vi "Confirm State Test.vi"(0 "GEA2 Reference In":refnum<k24>, 5 "Standalone?":bool, 7 "State":T1, 11 "Error In":errorcluster) -> (4 "GEA2 Reference Out":refnum<k24>, 6 "Pass/Fail?":bool, 15 "Error Out":errorcluster)   [LabVIEW 2016, in "Centauro.lvlib"]
uses:
  Projects/Centauro.lvlib
  Q:/Common/DLLs/GEA3/GeaCommunication.dll
  Common/DLLs/GEA3/GeaCommunication.dll
  type defs/Machine State.ctl
  Common/LabVIEW GEA2 Toolkit/LabVIEW_GEA2_Toolkit.lvlibp/type defs/Source_Destination.ctl
  Common/LabVIEW GEA2 Toolkit/LabVIEW_GEA2_Toolkit.lvlibp/type defs/ERD Read Data In.ctl
  Common/LabVIEW GEA2 Toolkit/LabVIEW_GEA2_Toolkit.lvlibp/type defs/Data Type.ctl
  Common/LabVIEW GEA2 Toolkit/LabVIEW_GEA2_Toolkit.lvlibp
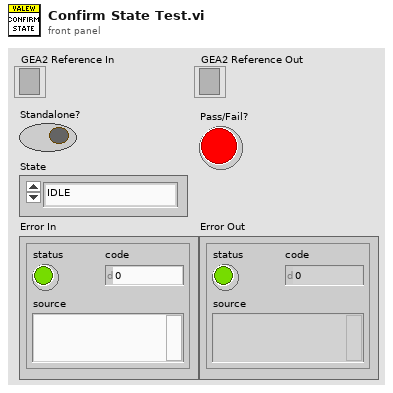
[diagram p1: front panel]
types:
  T1 = typedef "Centauro.lvlib/Machine State.ctl" = enum16{"IDLE", "STANDBY", "DELAY", "RUN", "PAUSE", "DELAY PAUSE", "EOC"}
  T2 = typedef "LabVIEW_GEA2_Toolkit.lvlibp/ERD Read Data In.ctl" = cluster{"ERD Number":u16, "Data Type":T3}
  T3 = typedef "LabVIEW_GEA2_Toolkit.lvlibp/Data Type.ctl" = enum16{"string", "boolean", "uint8_t", "uint16_t", "uint32_t", "uint64_t", "int8_t", "int16_t", "int32_t", "int64_t"}
  T4 = typedef "LabVIEW_GEA2_Toolkit.lvlibp/Source_Destination.ctl" = cluster{"Source":u8, "Destination":u8}
  T5 = typedef "LabVIEW_GEA2_Toolkit.lvlibp/ERD Read Data Out.ctl" = cluster{"ERD Number":u16, "Data":string}
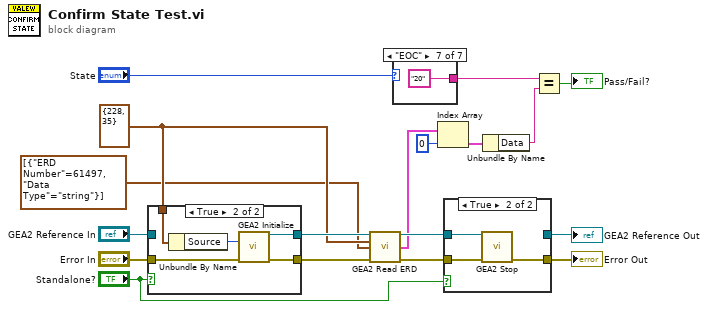
[diagram p0: block diagram]
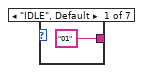
[diagram p2: hidden frame]
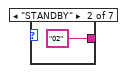
[diagram p3: hidden frame]
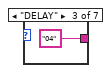
[diagram p4: hidden frame]
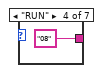
[diagram p5: hidden frame]
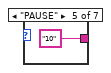
[diagram p6: hidden frame]
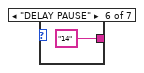
[diagram p7: hidden frame]
diagram:
  w10 = T4 {"Source"=228, "Destination"=35} ("GEA Inputs")
  n1 = case shown="True" "Standalone?" {
    tunnel: "Error In" -> [w19 w25]
    tunnel: [w19 w24] -> w14
    tunnel: "GEA2 Reference In" -> [w20 _]
    tunnel: [w20 w23] -> w12
    tunnel: w10 -> [_ w21]
    frame False {
    }
    frame True {
      n2 = Unbundle By Name(w21) -> ("Source"=w22:u8)
      n3 = call "GEA2 Initialize.vi"("Source Address"=w22, "error in"=w25) -> ("GEA2 Reference Out"=w23:refnum<k24>, "error out"=w24:errorcluster)  [unwired: 11 in, 1 out]
    }
  }
  n4 = call "GEA2 Read ERD.vi"("GEA2 Reference In"=w12, "GEA Inputs"=w10, "Read ERD List"=T2[] [{"ERD Number"=61497, "Data Type"=enum."string"}], "Error In"=w14) -> ("GEA2 Reference Out"=w11:refnum<k24>, "ERD Data Out"=w8:T5[], "Error Out"=w13:errorcluster)  [unwired: 8 in, 1 out]
  n5 = case shown="\"EOC\"" "State" {
    tunnel: ["01" "02" "04" "08" "10" "14" "20"] -> w3
    frame "IDLE", Default {
    }
    frame "STANDBY" {
    }
    frame "DELAY" {
    }
    frame "RUN" {
    }
    frame "PAUSE" {
    }
    frame "DELAY PAUSE" {
    }
    frame "EOC" {
    }
  }
  n6 = Index Array(array=w8, index=0) -> (element=w6:T5)
  n7 = case shown="True" "Standalone?" {
    tunnel: [w34 w37] -> w16
    tunnel: w13 -> [w34 w36]
    tunnel: w11 -> [w33 w35]
    tunnel: [w33 _] -> w1
    frame False {
    }
    frame True {
      n8 = call "GEA2 Stop.vi"("GEA2 Reference In"=w35, "Error In"=w36) -> ("Error Out"=w37:errorcluster)  [unwired: 13 in]
    }
  }
  "Error Out" <- w16
  "GEA2 Reference Out" <- w1
  n9 = Unbundle By Name(w6) -> ("Data"=w5:string)
  n10 = Equal?(x=w3, y=w5) -> (x = y?=→"Pass/Fail?":bool)
